vi "query field.vi"(8 "error in (no error)":errorcluster, 11 "VISA session":refnum<visa-resource-name>) -> (0 "error out":errorcluster, 2 "Field reading":dbl[unit], 3 "dup VISA session":refnum<visa-resource-name>)   [LabVIEW 2017]
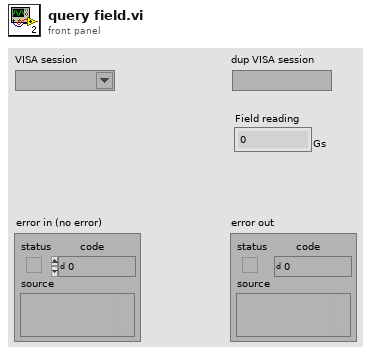
[diagram p1: front panel]
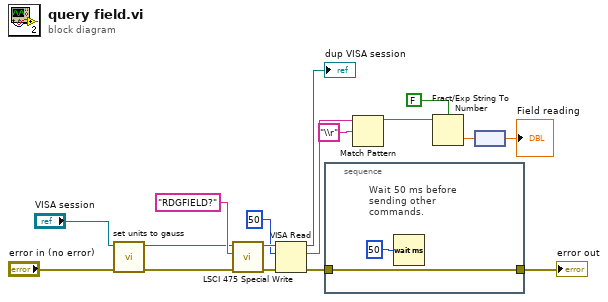
[diagram p0: block diagram]
diagram:
  n1 = call "set units to gauss.vi"("VISA session"="VISA session", "error in (no error)"="error in (no error)") -> ("dup VISA session"=w5:refnum<visa-resource-name>, "error out"=w3:errorcluster)  [unwired: 7 in]
  n2 = call "LSCI 475 Special Write.vi"("error in (no error)"=w3, "Write Buffer (\"\")"="RDGFIELD?", "VISA session"=w5) -> ("error out"=w14:errorcluster, "dup VISA session"=w15:refnum<visa-resource-name>)  [unwired: 6 in, 1 out]
  n3 = VISA Read(VISA resource name=w15, byte count=u32 50, error in (no error)=w14) -> (VISA resource name out=→"dup VISA session":refnum<visa-resource-name>, read buffer=w12:string, error out=w8:errorcluster)  [unwired: 1 out]
  n4 = stacked-sequence {
    tunnel: w8 -> [w18]
    tunnel: [w18] -> w7
    frame #0 {
      # "Wait 50 ms before\nsending other\ncommands."
      n5 = Wait (ms)(milliseconds to wait=u32 50) -> ()  [unwired: 1 out]
    }
  }
  "error out" <- w7
  n6 = Match Pattern(string=w12, regular expression="\\r") -> (before substring=w10:string)  [unwired: 1 in, 3 out]
  n7 = Fract/Exp String To Number(use system decimal point (T)=FALSE, string=w10) -> (number=w2:dbl)  [unwired: 2 in, 1 out]
  n8 = node(w2) -> (→"Field reading":dbl[unit])
